vi "Seleccionar producto.vi"(11 "PRODUCTOS EN Array":T1(array[cluster])) -> (3 "Array":string[][](array[string]))   [LabVIEW 2020]
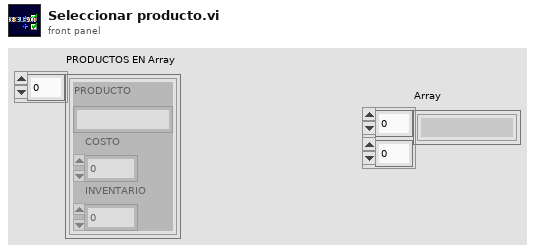
[diagram p1: front panel]
types:
  T1 = cluster{"PRODUCTO":string, "COSTO":dbl, "INVENTARIO":dbl}[]
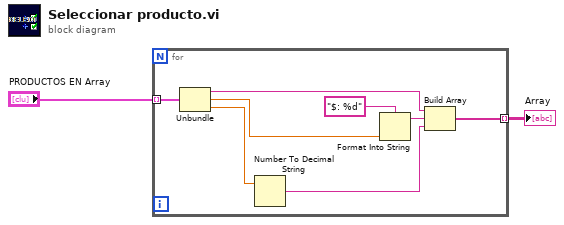
[diagram p0: block diagram]
diagram:
  n1 = for {
    tunnel: "PRODUCTOS EN Array" -> [w10] mode=indexing
    tunnel: [w3] -> w1 mode=indexing
    n2 = Unbundle "Unbundle"(w10) -> ("PRODUCTO"=w7:string, "COSTO"=w8:dbl, "INVENTARIO"=w6:dbl)
    n3 = Number To Decimal String(number=w6) -> (decimal integer string=w5:string)  [unwired: 1 in]
    n4 = Format Into String(format string="$: %d", w8) -> (resulting string=w4:string)  [unwired: 2 in, 1 out]
    n5 = Build Array "Build Array"(w7, w4, w5) -> (w3:string[])
  }
  "Array" <- w1
